vi "UserInParse.vi"(2 "User Input":bool[](array[boolean])) -> (6 "Filename":string[](array[string]), 7 "Measurement":string[](array[string]))   [LabVIEW 2018]
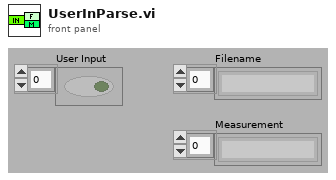
[diagram p1: front panel]
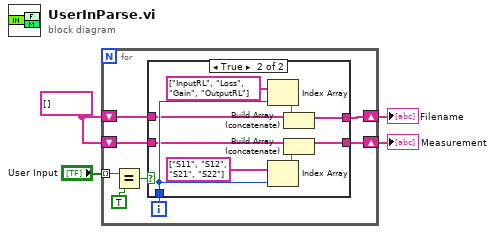
[diagram p0: block diagram]
diagram:
  w2 = string[] []
  n1 = for {
    tunnel: "User Input" -> [w10] mode=indexing
    shift-right: [w5] -> w3
    shift-left: w2 -> [w7]
    shift-right: [w6] -> w4
    shift-left: w2 -> [w8]
    i -> [w12]
    n2 = Equal?(x=w10, y=TRUE) -> (x = y?=w9:bool)
    n3 = case shown="True" w9 {
      tunnel: w12 -> [_ w23]
      tunnel: w8 -> [w14 w19]
      tunnel: w7 -> [w13 w17]
      tunnel: [w14 w18] -> w6
      tunnel: [w13 w15] -> w5
      frame False {
      }
      frame True {
        n4 = Index Array(array=string[] ["InputRL", "Loss", "Gain", "OutputRL"] ("Filename"), index=w23) -> (element=w16:string)
        n5 = Index Array(array=string[] ["S11", "S12", "S21", "S22"], index=w23) -> (element=w20:string)
        n6 = Build Array (concatenate)(w17, w16) -> (w15:string[])
        n7 = Build Array (concatenate)(w19, w20) -> (w18:string[])
      }
    }
  }
  "Filename" <- w3
  "Measurement" <- w4
